vi "Initialize Routing and Faulting Engine.vi"(8 "error in (no error)":errorcluster, 9 "Device Inputs FIFO":refnum<k33>, 10 "Device Outputs FIFO":refnum<k33>, 11 "Device Ref in":T12 format="%.0x") -> (0 "error out":errorcluster, 2 "Engine Data":T1, 3 "Device Ref out":T12 format="%.0x")   [LabVIEW 2017, in "Routing and Faulting Engine.lvlib"]
uses:
  Routing and Faulting Engine.lvlib
  <vilib>/NI Veristand/Custom Device API/Custom Device Item Ref.ctl
  Engine Data.ctl
  Includes/CDMessaging.lvlibp/Producer/Abstract Producer/Abstract Producer.lvclass
  Shared/Compiled.Settings.ctl
  Shared/Communication Configuration.ctl
  Shared/Routing and Faulting Configuration.ctl
  Shared/Routing Channel Configuration.ctl
  Shared/Value-Connections Map.ctl
  Shared/Connection.ctl
  Shared/Alias Mapping.ctl
  Shared/FIFO Indices.ctl
  Device Inputs.ctl
  Device Outputs.ctl
  Device FIFOs.ctl
  Shared/Constants.vi
  <vilib>/NI Veristand/Custom Device API/Get Item Property (Variant).vi
  Shared/Routing and Faulting Shared.lvlib
  <vilib>/NI Veristand/Custom Device API/Custom Device API.lvlib
  Includes/CDMessaging.lvlibp/Message/Abstract Message/Abstract Message.lvclass
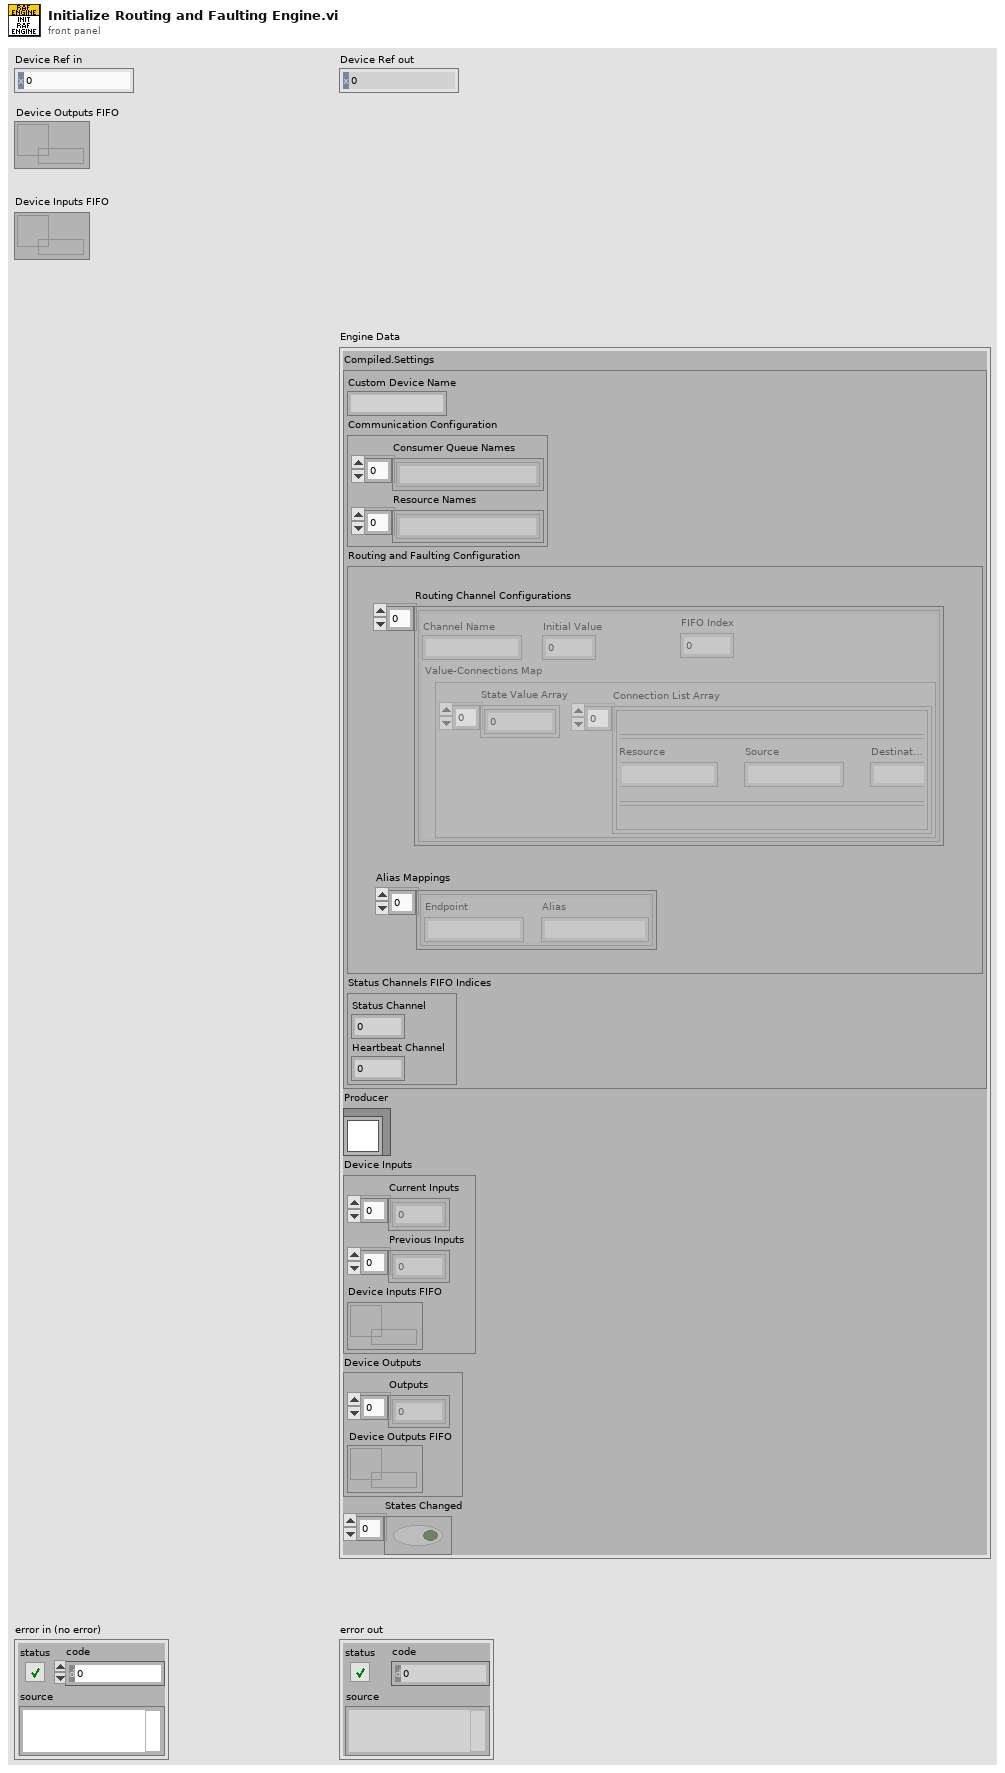
[diagram p1: front panel]
types:
  T1 = typedef "Routing and Faulting Engine.lvlib/Engine Data.ctl" = cluster{"Compiled.Settings":T2, "Producer":refnum<class "Abstract Producer.lvclass">, "Device Inputs":T10, "Device Outputs":T11, "States Changed":bool[]}
  T2 = typedef "Routing and Faulting Shared.lvlib/Compiled.Settings.ctl" = cluster{"Custom Device Name":string, "Communication Configuration":T3, "Routing and Faulting Configuration":T4, "Status Channels FIFO Indices":T9}
  T3 = typedef "Routing and Faulting Shared.lvlib/Communication Configuration.ctl" = cluster{"Consumer Queue Names":string[], "Resource Names":string[]}
  T4 = typedef "Routing and Faulting Shared.lvlib/Routing and Faulting Configuration.ctl" = cluster{"Routing Channel Configurations":T5[], "Alias Mappings":T8[]}
  T5 = typedef "Routing and Faulting Shared.lvlib/Routing Channel Configuration.ctl" = cluster{"Channel Name":string, "Initial Value":dbl, "FIFO Index":i32, "Value-Connections Map":T6}
  T6 = typedef "Routing and Faulting Shared.lvlib/Value-Connections Map.ctl" = cluster{"State Value Array":i32[], "Connection List Array":cluster{"Connection List":T7[]}[]}
  T7 = typedef "Routing and Faulting Shared.lvlib/Connection.ctl" = cluster{"Resource":string, "Source":string, "Destination":string}
  T8 = typedef "Routing and Faulting Shared.lvlib/Alias Mapping.ctl" = cluster{"Endpoint":string, "Alias":string}
  T9 = typedef "Routing and Faulting Shared.lvlib/FIFO Indices.ctl" = cluster{"Status Channel":i32, "Heartbeat Channel":i32}
  T10 = typedef "Routing and Faulting Engine.lvlib/Device Inputs.ctl" = cluster{"Current Inputs":dbl[], "Previous Inputs":dbl[], "Device Inputs FIFO":refnum<k33>}
  T11 = typedef "Routing and Faulting Engine.lvlib/Device Outputs.ctl" = cluster{"Outputs":dbl[], "Device Outputs FIFO":refnum<k33>}
  T12 = typedef "Custom Device API.lvlib/Custom Device Item Ref.ctl" = u64
  T13 = typedef "Routing and Faulting Engine.lvlib/Device FIFOs.ctl" = cluster{"Device Inputs FIFO":refnum<k33>, "Device Outputs FIFO":refnum<k33>}
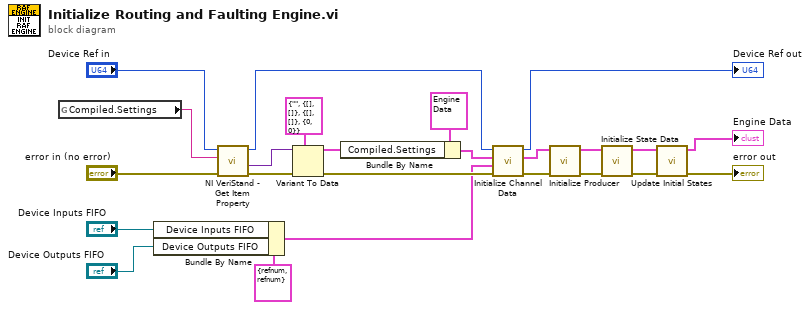
[diagram p0: block diagram]
diagram:
  n1 = global read "Constants.vi" "Compiled.Settings"() -> (w24:string)
  n2 = Bundle By Name(cluster=T13 {"Device Inputs FIFO"=refnum, "Device Outputs FIFO"=refnum} ("Device FIFOs"), "Device Inputs FIFO"="Device Inputs FIFO", "Device Outputs FIFO"="Device Outputs FIFO") -> (w8:T13)
  n3 = call-poly <vilib>:"NI VeriStand - Get Item Property.vi"("error in (no error)"="error in (no error)", "Property Name"=w24, "Item Ref in"="Device Ref in") -> ("error out"=w22:errorcluster, "Value"=w21:variant, "Item Ref out"=w14:T12)  [unwired: 5 in, 1 out]
  n4 = Variant To Data(error in=w22, type=T2 {"Custom Device Name"="", "Communication Configuration"={"Consumer Queue Names"=[], "Resource Names"=[]}, "Routing and Faulting Configuration"={"Routing Channel Configurations"=[], "Alias Mappings"=[]}, "Status Channels FIFO Indices"={"Status Channel"=0, "Heartbeat Channel"=0}} ("Compiled.Settings"), Variant=w21) -> (data=w17:T2, error out=w19:errorcluster)
  n5 = Bundle By Name(cluster=T1 {"Compiled.Settings"={"Custom Device Name"="", "Communication Configuration"={"Consumer Queue Names"=[], "Resource Names"=[]}, "Routing and Faulting Configuration"={"Routing Channel Configurations"=[], "Alias Mappings"=[]}, "Status Channels FIFO Indices"={"Status Channel"=0, "Heartbeat Channel"=0}}, "Producer"=refnum, "Device Inputs"={"Current Inputs"=[], "Previous Inputs"=[], "Device Inputs FIFO"=refnum}, "Device Outputs"={"Outputs"=[], "Device Outputs FIFO"=refnum}, "States Changed"=[]} ("Engine Data"), "Compiled.Settings"=w17) -> (w16:T1)
  n6 = call "Initialize Channel Data.vi"("error in (no error)"=w19, "FIFOs"=w8, "Engine Data in"=w16, "Device Ref in"=w14) -> ("error out"=w12:errorcluster, "Engine Data out"=w6:T1, "Device Ref out"=→"Device Ref out":T12)  [unwired: 5 in]
  n7 = call "Initialize Producer.vi"("error in (no error)"=w12, "Engine Data in"=w6) -> ("error out"=w7:errorcluster, "Engine Data out"=w5:T1)  [unwired: 8 in]
  n8 = call "Initialize State Data.vi"("error in (no error)"=w7, "Engine Data in"=w5) -> ("error out"=w4:errorcluster, "Engine Data out"=w2:T1)  [unwired: 8 in]
  n9 = call "Update Initial States.vi"("error in (no error)"=w4, "Engine Data in"=w2) -> ("error out"=→"error out":errorcluster, "Engine Data out"=→"Engine Data":T1)  [unwired: 8 in]
